vi "Initialize.vi"(8 "Error In":errorcluster, 11 "VI Path":path) -> (0 "Error Out":errorcluster, 1 "ABLE Configuration":T1, 2 "ABLE Data Structures":T7, 3 "Action Queues":T8)   [LabVIEW 2012]
uses:
  ActionQueues.ctl
  UIActionQueueElement.ctl
  UIAction.ctl
  HardwareActionQueueElement.ctl
  HardwareAction.ctl
  ExperimentActionQueueElement.ctl
  ExperimentAction.ctl
  AlarmQueueElement.ctl
  AlarmAction.ctl
  ABLEDataStructures.ctl
  HardwareDisplayData.ctl
  BPM.ctl
  ExperimentHardwareData.ctl
  ExperimentData.ctl
  AlarmData.ctl
  AlarmDatum.ctl
  ABLEConfiguration.ctl
  DisplayConfiguration.ctl
  FolderConfiguration.ctl
  AlarmsConfiguration.ctl
  Keithley6485Configuration.ctl
  Keithley6482Configuration.ctl
  libs/LV-Utilities/LV-Utilities.lvlib
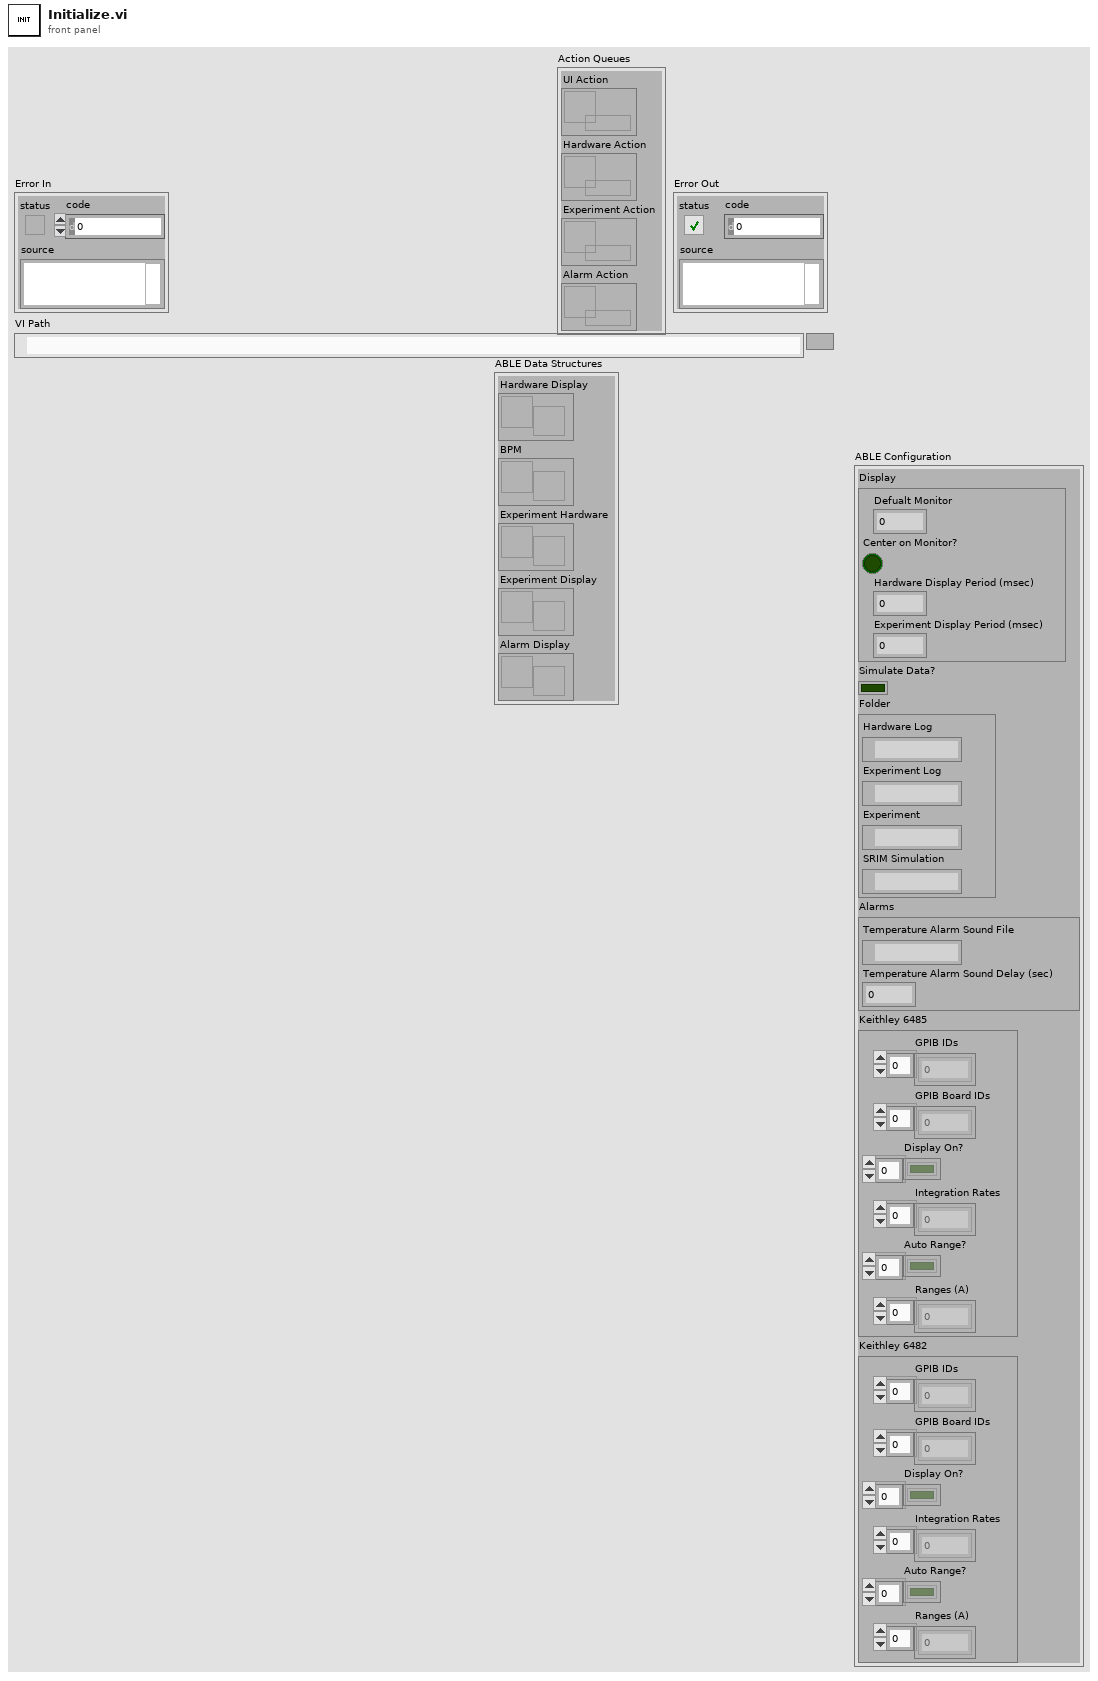
[diagram p1: front panel]
types:
  T1 = typedef "ABLEConfiguration.ctl" = cluster{"Display":T2, "Simulate Data?":bool, "Folder":T3, "Alarms":T4, "Keithley 6485":T5, "Keithley 6482":T6}
  T2 = typedef "DisplayConfiguration.ctl" = cluster{"Defualt Monitor":u16, "Center on Monitor?":bool, "Hardware Display Period (msec)":u32, "Experiment Display Period (msec)":u32}
  T3 = typedef "FolderConfiguration.ctl" = cluster{"Hardware Log":path, "Experiment Log":path, "Experiment":path, "SRIM Simulation":path}
  T4 = typedef "AlarmsConfiguration.ctl" = cluster{"Temperature Alarm Sound File":path, "Temperature Alarm Sound Delay (sec)":dbl}
  T5 = typedef "Keithley6485Configuration.ctl" = cluster{"GPIB IDs":u8[], "GPIB Board IDs":u8[], "Display On?":bool[], "Integration Rates":dbl[], "Auto Range?":bool[], "Ranges (A)":dbl[]}
  T6 = typedef "Keithley6482Configuration.ctl" = cluster{"GPIB IDs":u8[], "GPIB Board IDs":u8[], "Display On?":bool[], "Integration Rates":dbl[], "Auto Range?":bool[], "Ranges (A)":dbl[]}
  T7 = typedef "ABLEDataStructures.ctl" = cluster{"Hardware Display":refnum<notifier>, "BPM":refnum<notifier>, "Experiment Hardware":refnum<notifier>, "Experiment Display":refnum<notifier>, "Alarm Display":refnum<notifier>}
  T8 = typedef "ActionQueues.ctl" = cluster{"UI Action":refnum<queue>, "Hardware Action":refnum<queue>, "Experiment Action":refnum<queue>, "Alarm Action":refnum<queue>}
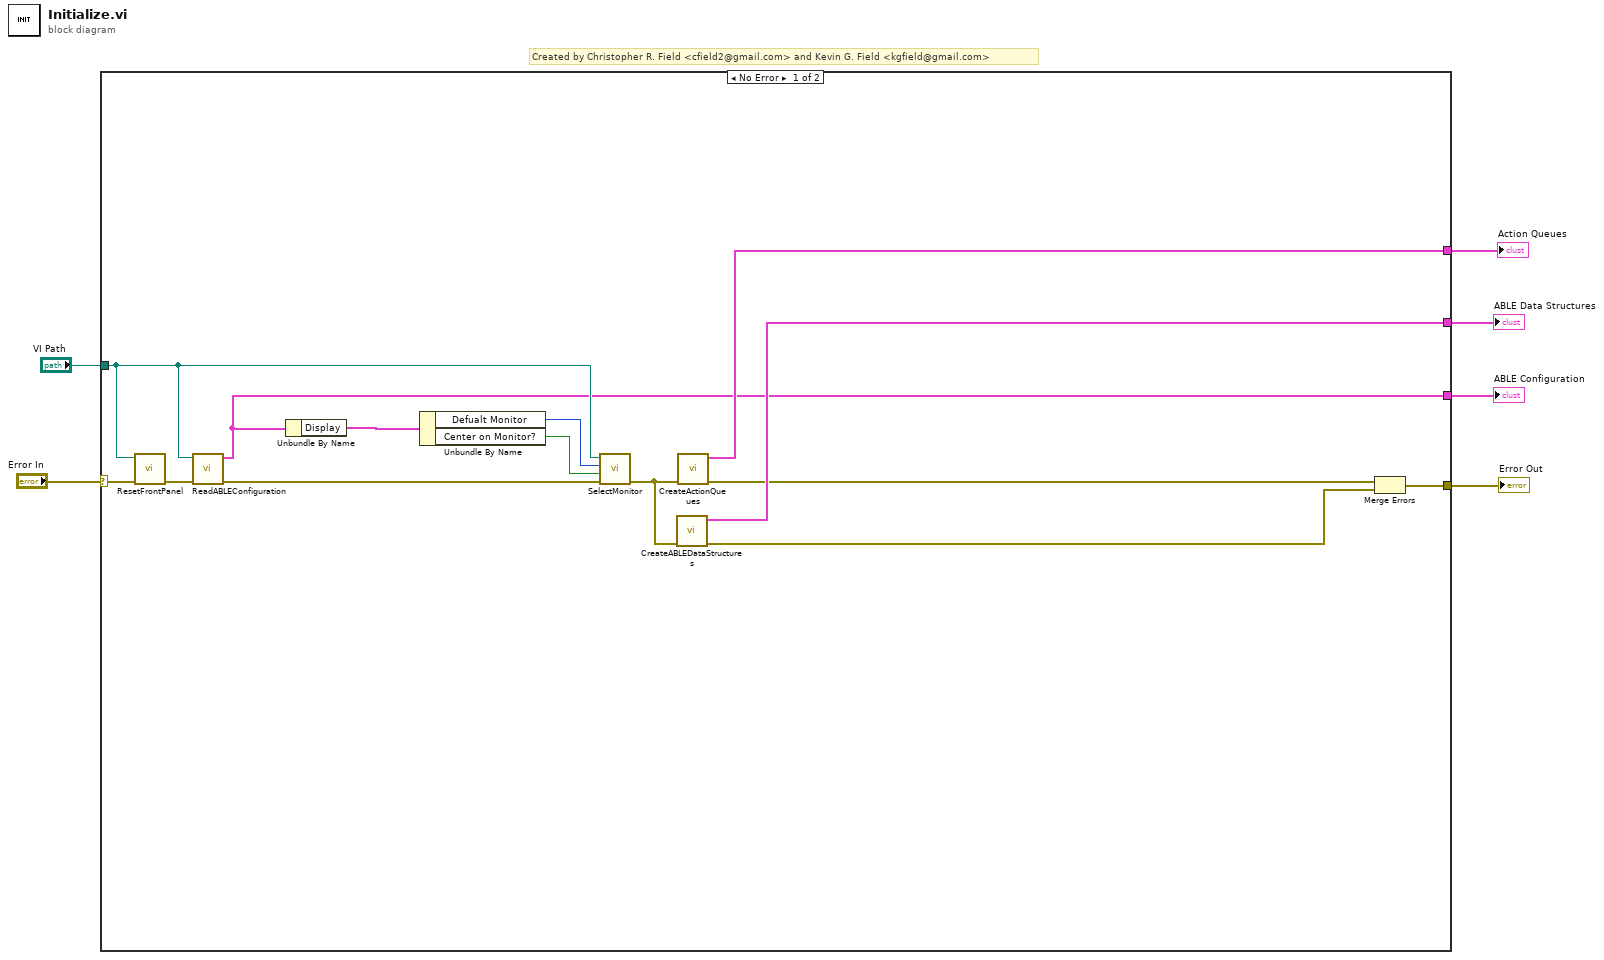
[diagram p0: block diagram]
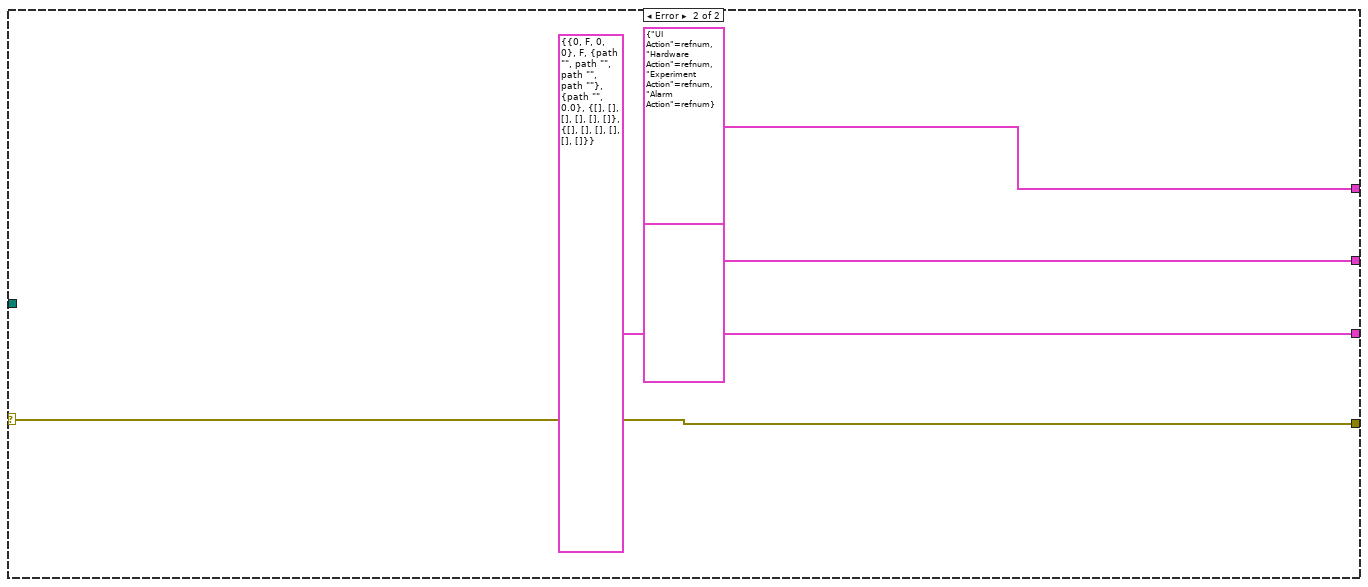
[diagram p2: hidden frame]
diagram:
  # "Created by Christopher R. Field <cfield2@gmail.com> and Kevin G. Field <kgfield@gmail.com>"
  n1 = case shown="No Error" "Error In" {
    selector: "Error In" -> [w15 w24]
    tunnel: [w20 T8 {"UI Action"=refnum, "Hardware Action"=refnum, "Experiment Action"=refnum, "Alarm Action"=refnum} ("Message Queues")] -> w6
    tunnel: [w17 w24] -> w5
    tunnel: "VI Path" -> [w13 _]
    tunnel: [w19 T7 {"Hardware Display"=refnum, "BPM"=refnum, "Experiment Hardware"=refnum, "Experiment Display"=refnum, "Alarm Display"=refnum} ("Data Communication Structures")] -> w2
    tunnel: [w10 T1 {"Display"={"Defualt Monitor"=0, "Center on Monitor?"=FALSE, "Hardware Display Period (msec)"=0, "Experiment Display Period (msec)"=0}, "Simulate Data?"=FALSE, "Folder"={"Hardware Log"=path "", "Experiment Log"=path "", "Experiment"=path "", "SRIM Simulation"=path ""}, "Alarms"={"Temperature Alarm Sound File"=path "", "Temperature Alarm Sound Delay (sec)"=0.0}, "Keithley 6485"={"GPIB IDs"=[], "GPIB Board IDs"=[], "Display On?"=[], "Integration Rates"=[], "Auto Range?"=[], "Ranges (A)"=[]}, "Keithley 6482"={"GPIB IDs"=[], "GPIB Board IDs"=[], "Display On?"=[], "Integration Rates"=[], "Auto Range?"=[], "Ranges (A)"=[]}} ("ABLE Configuration")] -> w1
    frame No Error {
      n2 = call "ResetFrontPanel.vi"("Error In"=w15, "VI Path"=w13) -> ("Error Out"=w14:errorcluster)  [unwired: 9 in]
      n3 = call "ReadABLEConfiguration.vi"("Error In"=w14, "VI Path"=w13) -> ("Error Out"=w12:errorcluster, "ABLE Configuration"=w10:T1)  [unwired: 8 in]
      n4 = Unbundle By Name(w10) -> ("Display"=w9:T2)
      n5 = Unbundle By Name(w9) -> ("Defualt Monitor"=w8:u16, "Center on Monitor?"=w7:bool)
      n6 = call "SelectMonitor.vi"("Error In"=w12, "Center?"=w7, "Monitor (0=primary)"=w8, "VI Path"=w13) -> ("Error out"=w11:errorcluster)  [unwired: 7 in]
      n7 = call "CreateABLEDataStructures.vi"("Error In"=w11) -> ("Error Out"=w16:errorcluster, "ABLE Data Structures"=w19:T7)  [unwired: 9 in]
      n8 = call "CreateActionQueues.vi"("Error In"=w11) -> ("Error Out"=w18:errorcluster, "Action Queues"=w20:T8)  [unwired: 9 in]
      n9 = Merge Errors(w18, w16) -> (w17:errorcluster)
    }
    frame Error {
    }
  }
  "Action Queues" <- w6
  "Error Out" <- w5
  "ABLE Data Structures" <- w2
  "ABLE Configuration" <- w1
